vi "Read IConfigure.vi"(8 "error in (no error)":errorcluster, 11 "Fgen Base in":refnum<class "FGEN Base.lvclass">) -> (0 "error out":errorcluster, 2 "IConfigure":refnum<class "IConfigure.lvclass">, 3 "Fgen Base out":refnum<class "FGEN Base.lvclass">)   [LabVIEW 2023, in "FGEN.lvlib" / "FGEN Base.lvlib" / "FGEN Base.lvclass"]
uses:
  FGEN Base.lvclass
  Interfaces/IConfigure/IConfigure.lvclass
  FGEN Base.lvclass/FGEN Base.ctl
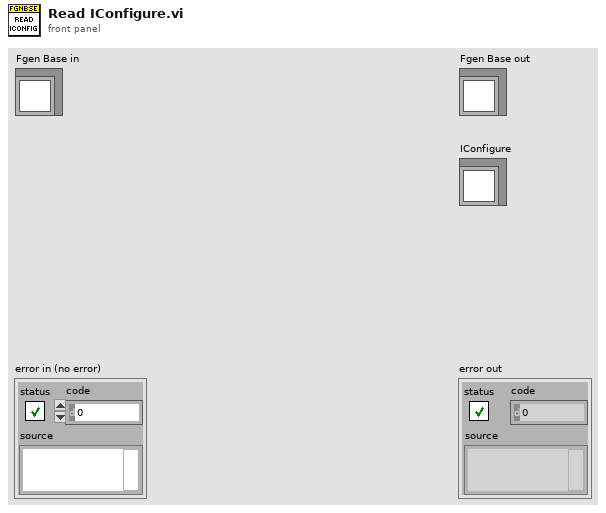
[diagram p1: front panel]
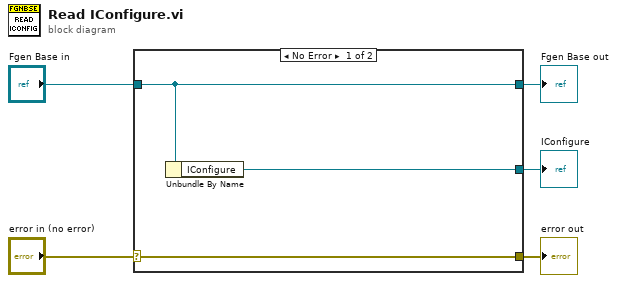
[diagram p0: block diagram]
diagram:
  n1 = case shown="No Error" "error in (no error)" {
    selector: "error in (no error)" -> [w8 w9]
    tunnel: [w8 w9] -> w4
    tunnel: [w7 w10] -> w2
    tunnel: "Fgen Base in" -> [w7 w10]
    tunnel: [w6 _] -> w1
    frame No Error {
      n2 = Unbundle By Name(w7) -> ("IConfigure"=w6:refnum<class "IConfigure.lvclass">)
    }
    frame Error {
    }
  }
  "error out" <- w4
  "Fgen Base out" <- w2
  "IConfigure" <- w1
